vi "meTEC_Check for Device Error.vi"(7 "TEC Configuration_IN":T1={"VISA resource name"="", "Device Address"=2}, 8 "error in (no error)":errorcluster) -> (0 "error out":errorcluster)   [LabVIEW 2010]
uses:
  TypeDefs/meTEC_Configuration.ctl
panel:
  # "--- Outputs ---"
  # "--- Inputs ---"
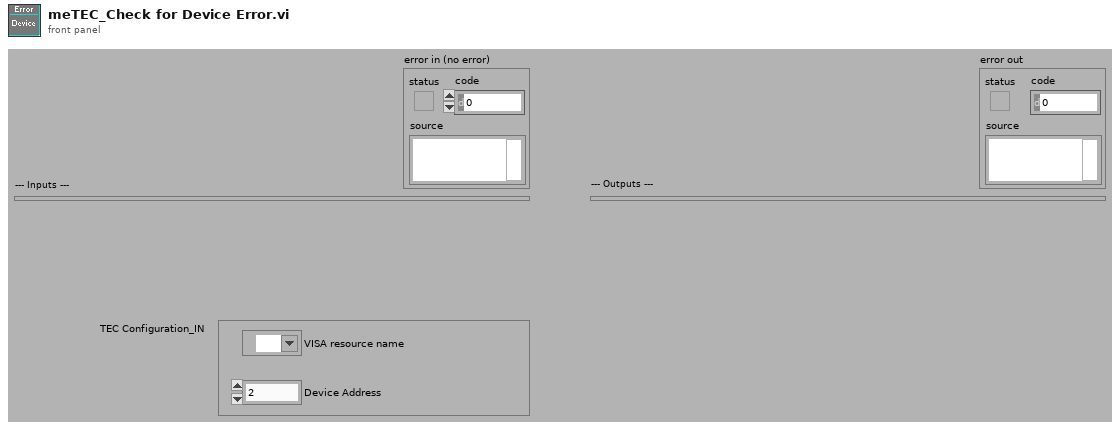
[diagram p1: front panel]
types:
  T1 = typedef "meTEC_Configuration.ctl" = cluster{"VISA resource name":refnum<visa-resource-name>, "Device Address":u16}
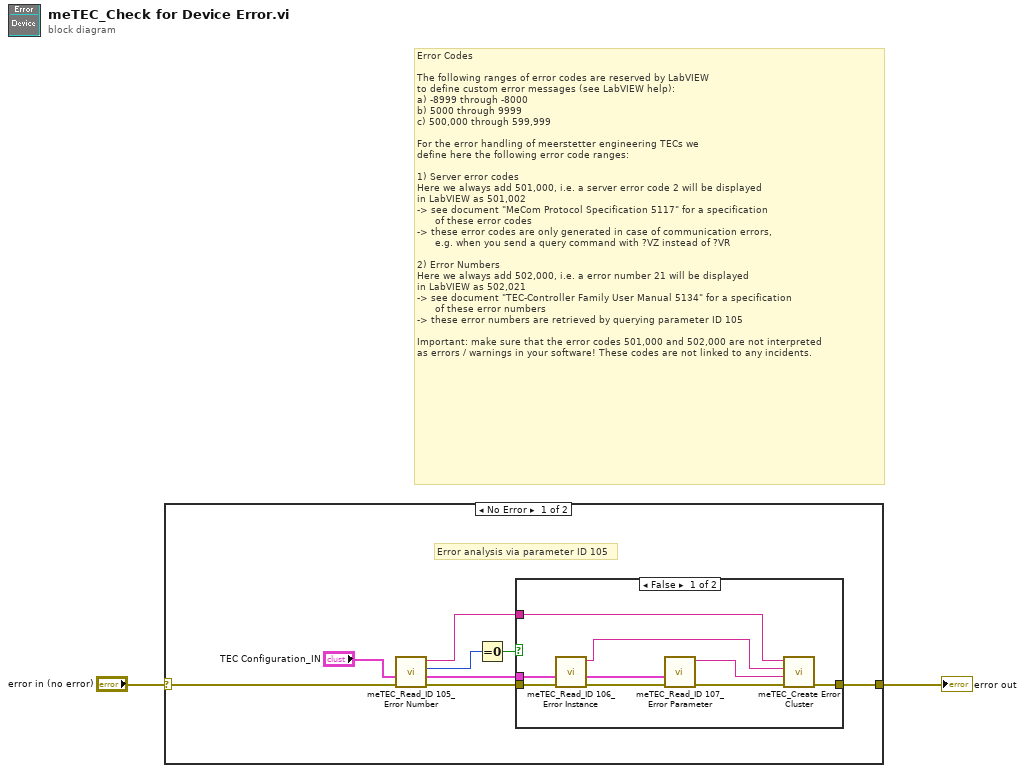
[diagram p0: block diagram]
diagram:
  # "Error Codes\n\nThe following ranges of error codes are reserved by LabVIEW\nto define custom error messages (see LabVIEW help):\na) -8999 through -8000 \nb) 5000 through 9999 \nc) 500,000 through 599,999\n\nFor the error handling of meerstetter engineering TECs we\ndefine here the following error code ranges:\n\n1) Server error codes\nHere we always add 501,000, i.e. a server error code 2 will be displayed\nin LabVIEW as 501,002\n-> see document \"MeCom Protocol Specification 5117\" for a specification \n      of these error codes\n-> these error codes are only generated in case of communication errors, \n      e.g. when you send a query command with ?VZ instead of ?VR \n\n2) Error Numbers\nHere we always add 502,000, i.e. a error number 21 will be displayed\nin LabVIEW as 502,021 \n-> see document \"TEC-Controller Family User Manual 5134\" for a specification \n      of these error numbers\n-> these error numbers are retrieved by querying parameter ID 105 \n\nImportant: make sure that the error codes 501,000 and 502,000 are not interpreted\nas errors / warnings in your software! These codes are not linked to any incidents."
  n1 = case shown="No Error" "error in (no error)" {
    selector: "error in (no error)" -> [w10 w21]
    tunnel: [w8 w21] -> w2
    frame No Error {
      # "Error analysis via parameter ID 105"
      n2 = call "meTEC_Read_ID 105_Error Number.vi"("error in (no error)"=w10, "TEC Configuration_IN"="TEC Configuration_IN") -> ("error out"=w7:errorcluster, "TEC Configuration_OUT"=w6:T1, "Error Number (ID 105) [I32]"=w4:i32, "Error Number (ID 105) [String]"=w3:string)  [unwired: 6 in]
      n3 = Equal To 0?(x=w4) -> (x = 0?=w5:bool)
      n4 = case shown="False" w5 {
        tunnel: w7 -> [w19 w20]
        tunnel: w6 -> [w17 _]
        tunnel: [w14 w20] -> w8
        tunnel: w3 -> [w11 _]
        frame False {
          n5 = call "meTEC_Read_ID 106_Error Instance.vi"("error in (no error)"=w19, "TEC Configuration_IN"=w17) -> ("error out"=w18:errorcluster, "TEC Configuration_OUT"=w16:T1, "Error Instance (ID 106) [String]"=w12:string)  [unwired: 6 in, 1 out]
          n6 = call "meTEC_Read_ID 107_Error Parameter.vi"("error in (no error)"=w18, "TEC Configuration_IN"=w16) -> ("error out"=w15:errorcluster, "Error Parameter (ID 107) [String]"=w13:string)  [unwired: 6 in, 2 out]
          n7 = call "meTEC_Create Error Cluster.vi"("error in (no error)"=w15, "Error Parameter"=w13, "Error Instance"=w12, "Error Number"=w11) -> ("error out"=w14:errorcluster)  [unwired: 7 in]
        }
        frame True {
        }
      }
    }
    frame Error {
    }
  }
  "error out" <- w2
